vi "AutoMode.vi"(8 "error in (no error)":errorcluster, 11 "AutoModeData":T1) -> (0 "error out":errorcluster)   [LabVIEW 2019, in "AutoMode.lvlib"]
uses:
  AutoMode.lvlib
  Cluster - AutoModeData.ctl
  MainController/Cluster - TestSettings.ctl
  MainController/Cluster - HardwareConfiguration.ctl
  MainController/Cluster - TestResults.ctl
  Cluster - AutoModeMessage.ctl
  Enum - AutoModeState.ctl
  MainController/Cluster - MainControllerMessage.ctl
  MainController/Enum - MainState.ctl
  support/User Event - Stop/User Event - Stop.lvlib
  MainController/MainController.lvlib
panel:
  in  "Manual Return To Zero":bool=TRUE
  in  "Dwell Time":dbl min=0.0 step=1.0 format="%.2f s"
  in  "Auto Increment":bool=TRUE
  in  "AutoGenerate":bool
  in  "Output Data Path":path
  in  "Goto Zero":bool
  in  "Zero Position":bool
  out "TravelForce":cluster{"Travel":dbl, "Force":dbl, "Work":dbl} {"Work" format="%.3f"; "Force" format="%.3f"; "Travel" format="%.3f"}
  in  "Applicator Prefix":string="Applicator Test"
  in  "Sample":u32=1
  in  "Winding Speed":dbl min=0.0 step=1.0 format="%.2f °/s"
  in  "Winding Distance":dbl min=0.0 step=1.0 format="%.2f °"
  out "TestRuntime":i64 format="%<%H:%M:%S>t"
  out "XY Graph":T5(graph)
  out "Waveform":dbl[][](graph) caption="Waveform Chart"
  out "Work":cluster{dbl[], "Real Matrix":dbl[]}[](graph)
  out "Running":bool
  # "Test Settings"
  # "Commands"
  # "DAQ I/O"
  # "Test Runtime"
  # "Travel (deg)"
  # "Force (N)"
  # "Work"
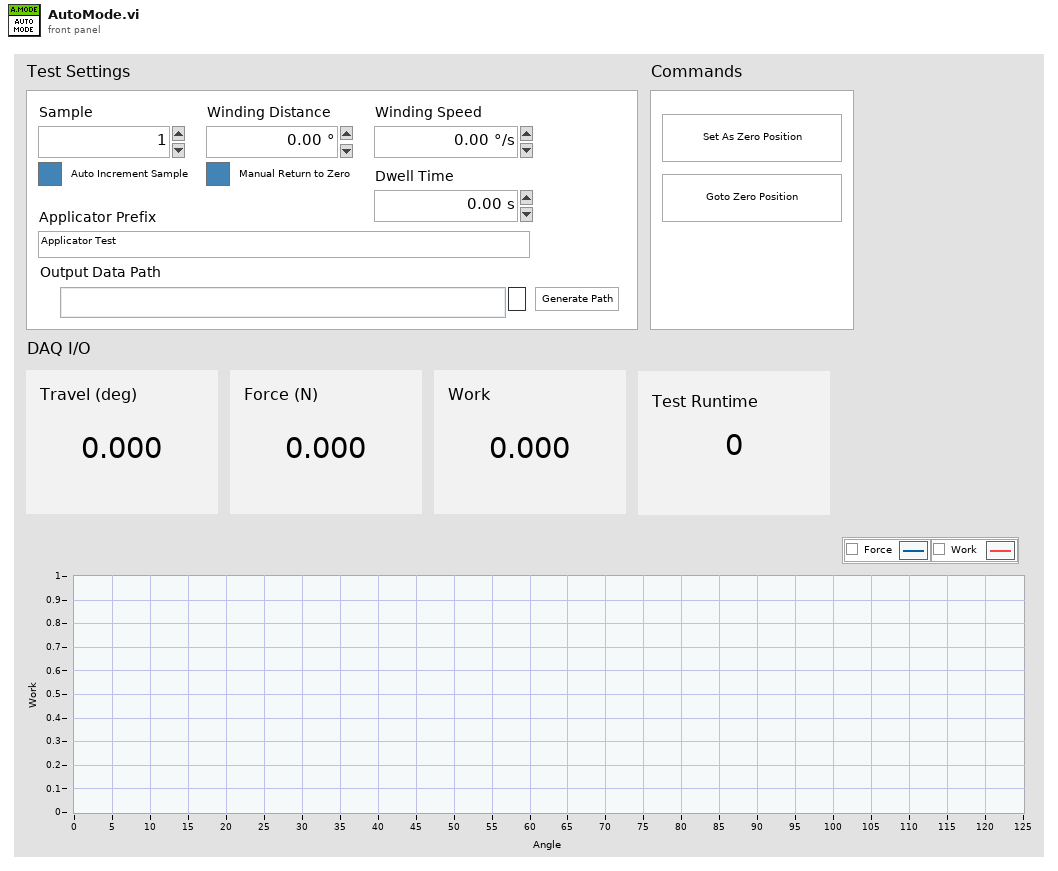
[diagram p1: front panel]
types:
  T1 = typedef "AutoMode.lvlib/Cluster - AutoModeData.ctl" = cluster{"DataDisplayQueue":refnum<queue>, "StepStartTime":timestamp, "TestSettings":T2, "Hardware Configuration":T3, "TestResults":T4, "ElapsedTime":dbl, "IsFirstSample":bool, "UIRefs":map{string, refnum<vi>}, "SelfQueue":refnum<queue>, "MainQueue":refnum<queue>}
  T2 = typedef "MainController.lvlib/Cluster - TestSettings.ctl" = cluster{"Sample":u32, "Applicator Prefix":string, "Winding Distance":dbl, "Winding Speed":dbl, "Dwell Time":dbl, "Auto Increment Sample":bool, "Output Data Path":path, "File Base Path":path, "Manual Return To Zero":bool}
  T3 = typedef "MainController.lvlib/Cluster - HardwareConfiguration.ctl" = cluster{"Mark10COM":refnum<visa-resource-name>, "IsConnected":bool}
  T4 = typedef "MainController.lvlib/Cluster - TestResults.ctl" = cluster{"AcquiredData":dbl[][], "TestStartTime":timestamp}
  T5 = cluster{"XY Graph":cluster{"X":dbl, "Y":dbl}[]}[]
  T6 = typedef "AutoMode.lvlib/Cluster - AutoModeMessage.ctl" = cluster{"Message":T7, "Data":variant}
  T7 = typedef "AutoMode.lvlib/Enum - AutoModeState.ctl" = enum16{"Initialize", "Idle", "UpdateConfig", "UpdateHWConfig", "BroadcastSettings", "Start", "CheckValidReportPath", "Winding", "WaitForWinding", "Unwind", "WaitForUnwind", "Stop", "Abort", "WriteDataToFile", "EventTriggered", "GenerateFilePath", "ZeroPosition", "GotoZero", "Error", "Exit"}
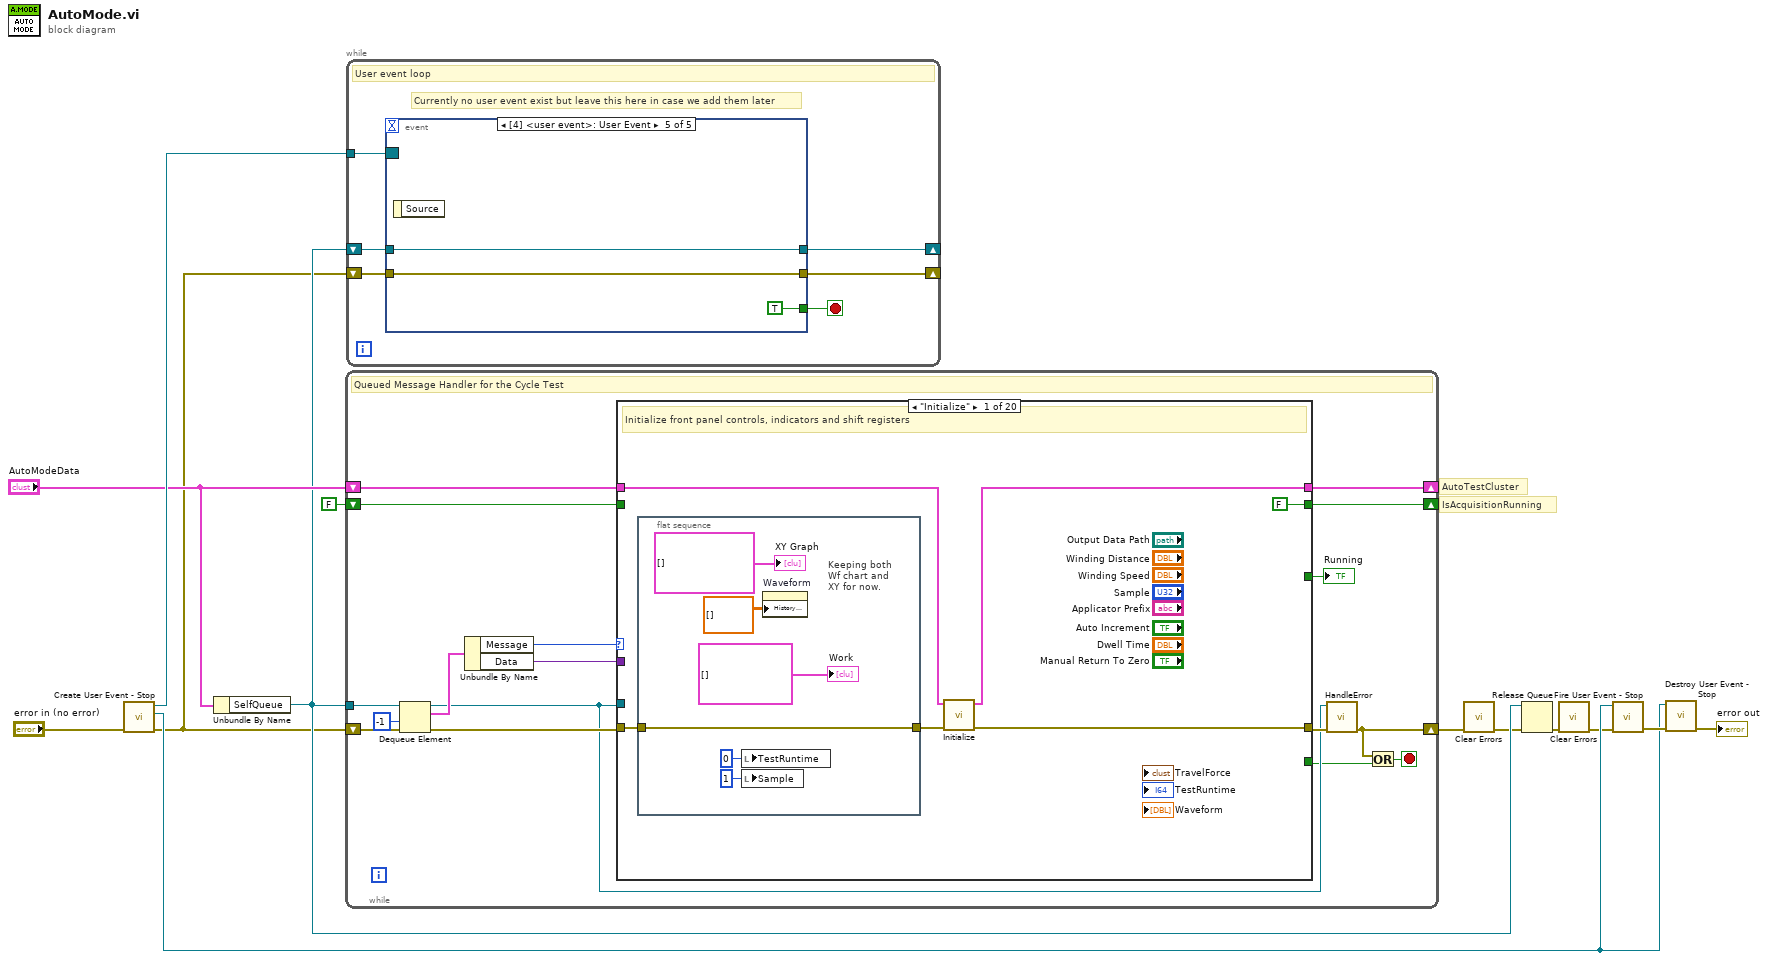
[diagram p0: block diagram]
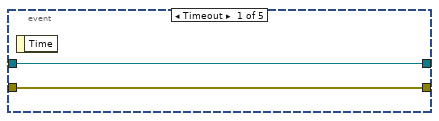
[diagram p2: hidden frame]
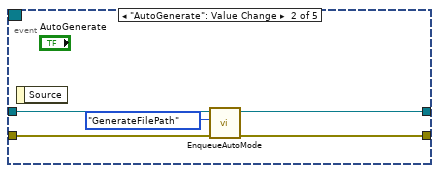
[diagram p3: hidden frame]
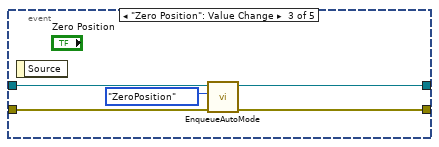
[diagram p4: hidden frame]
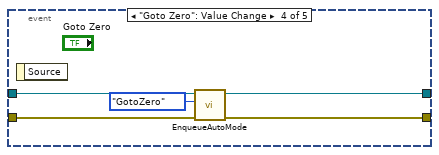
[diagram p5: hidden frame]
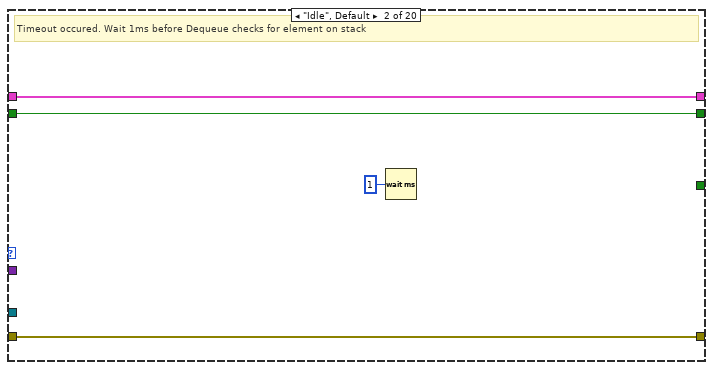
[diagram p6: hidden frame]
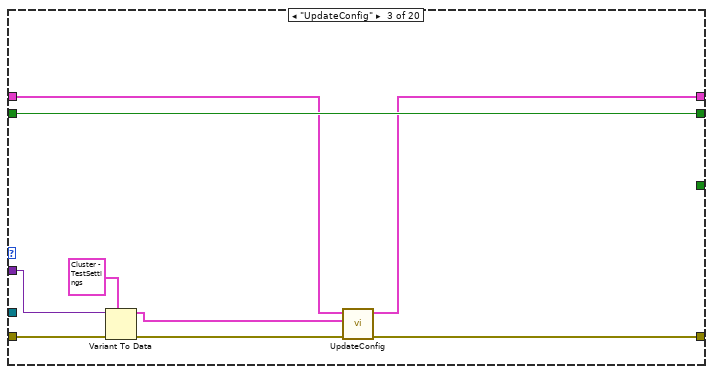
[diagram p7: hidden frame]
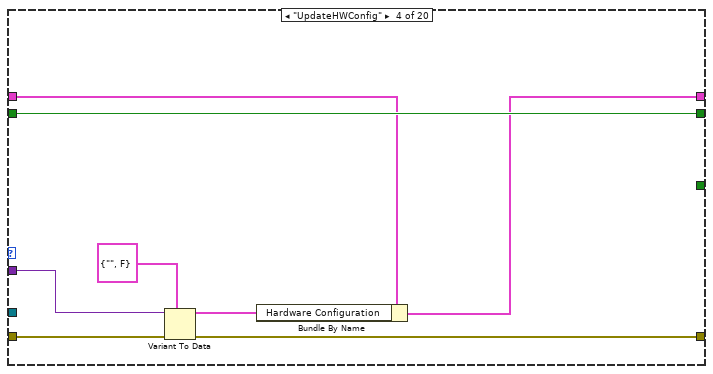
[diagram p8: hidden frame]
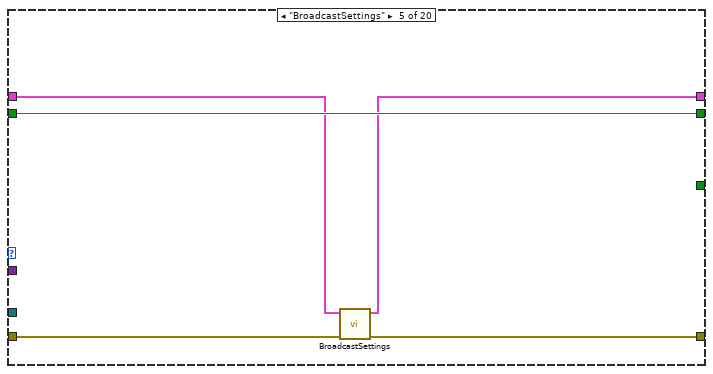
[diagram p9: hidden frame]
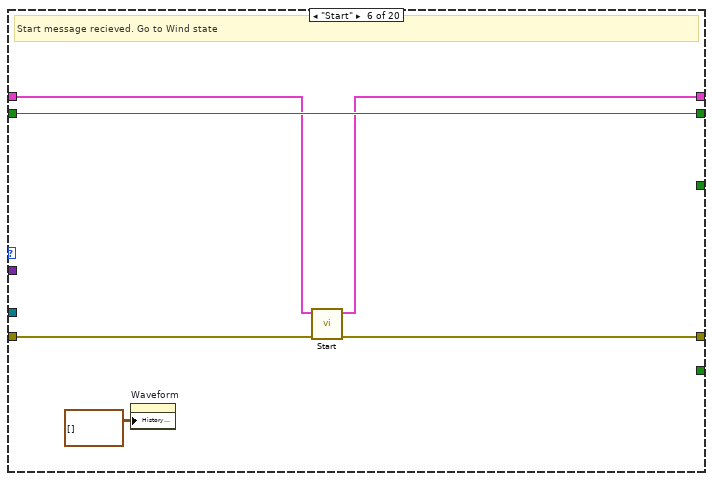
[diagram p10: hidden frame]
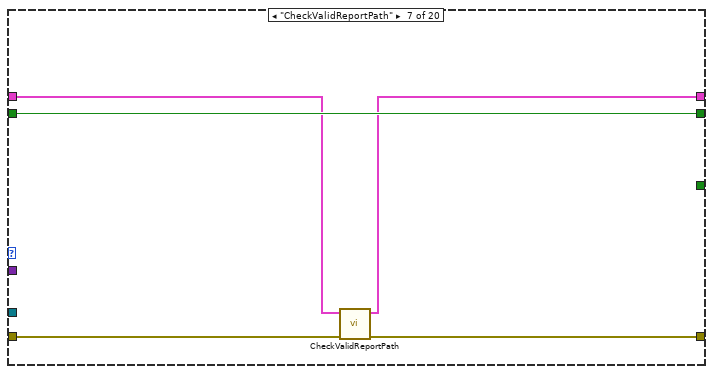
[diagram p11: hidden frame]
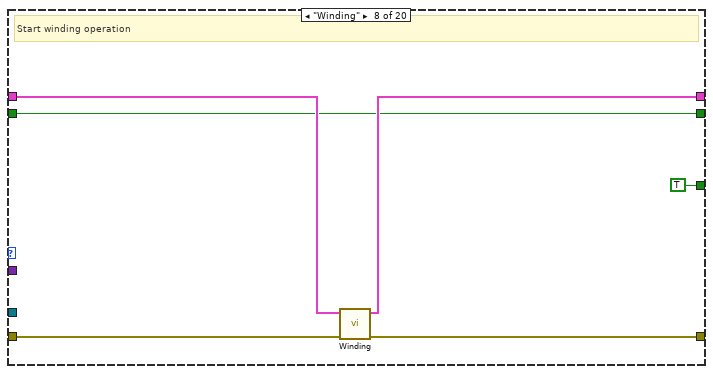
[diagram p12: hidden frame]
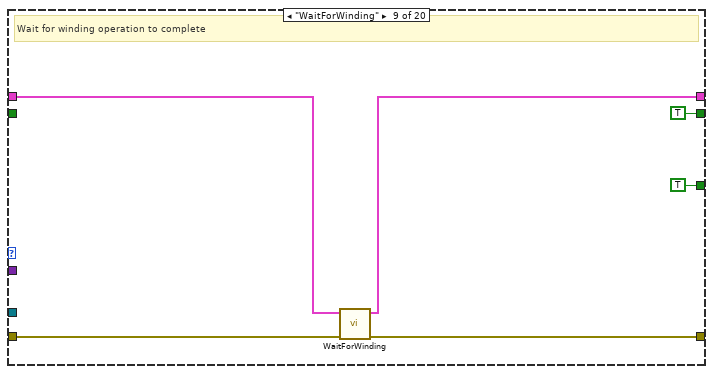
[diagram p13: hidden frame]
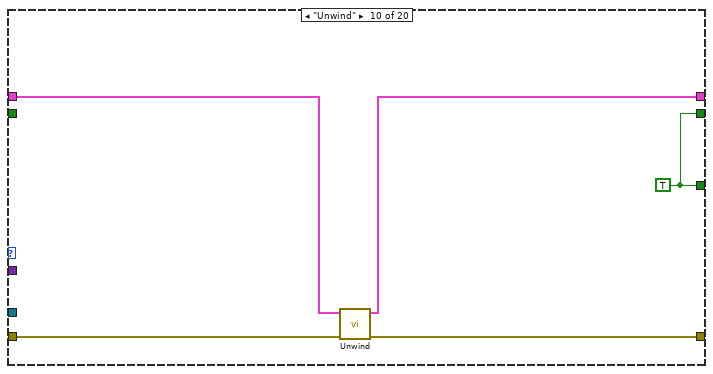
[diagram p14: hidden frame]
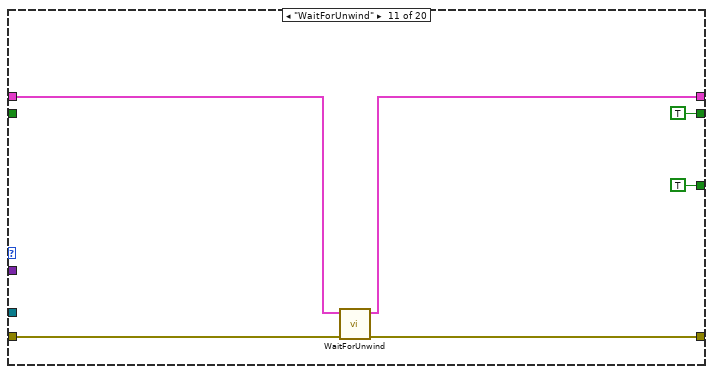
[diagram p15: hidden frame]
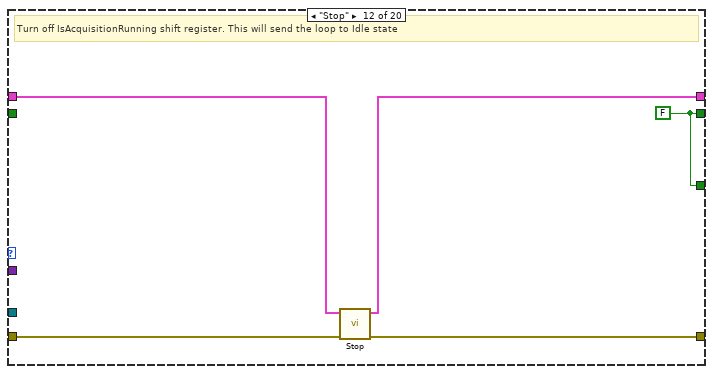
[diagram p16: hidden frame]
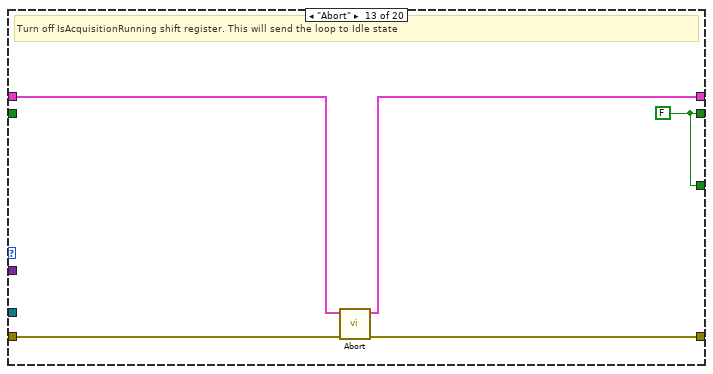
[diagram p17: hidden frame]
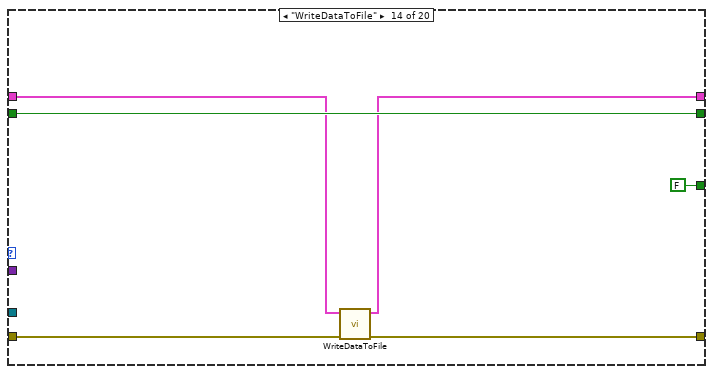
[diagram p18: hidden frame]
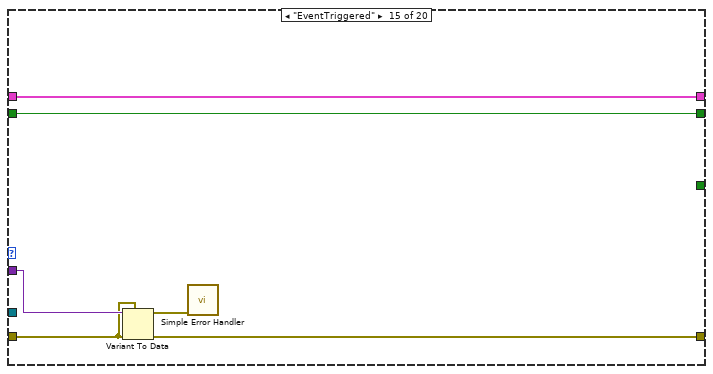
[diagram p19: hidden frame]
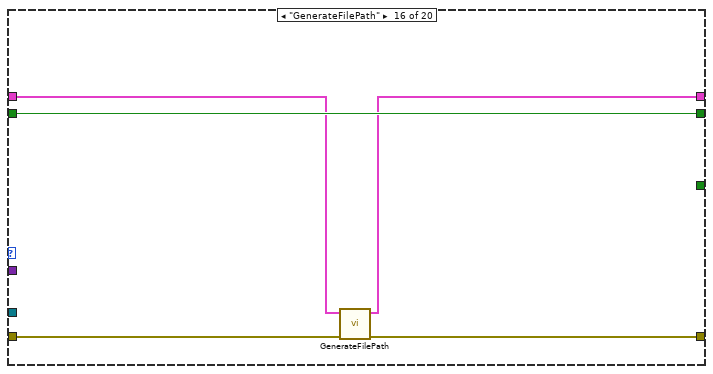
[diagram p20: hidden frame]
diagram:
  # "AutoTestCluster"
  # "IsAcquisitionRunning"
  n1 = call "Create User Event - Stop.vi"("error in (no error)"="error in (no error)") -> ("error out"=w3:errorcluster, "User Event - Stop"=w8:refnum<user-event>, "Stop Event Registration Refnum"=w12:refnum<event-registration>)  [unwired: 8 in]
  n2 = Unbundle By Name("AutoModeData") -> ("SelfQueue"=w4:refnum<queue>)
  n3 = while {
    tunnel: w4 -> [w29]
    shift-right: [w23] -> _
    shift-left: "AutoModeData" -> [w24]
    shift-right: [w21] -> _
    shift-left: FALSE -> [w20]
    shift-right: [w14] -> w13
    shift-left: w3 -> [w30]
    stop <- w15 stop-if-true
    # "Queued Message Handler for the Cycle Test"
    n4 = Dequeue Element(queue=w29, timeout in ms (-1)=-1, error in (no error)=w30) -> (queue out=w19:refnum<queue>, element=w28:T6, error out=w26:errorcluster)  [unwired: 1 out]
    n5 = Unbundle By Name(w28) -> ("Message"=w17:T7, "Data"=w25:variant)
    n6 = case shown="\"Initialize\"" w17 {
      tunnel: [w31 w43 w49 w61 w66 w71 w77 w83 w88 w94 w99 w105 w110 w115 w122 w127 w132 w137 w142 w153] -> w27
      tunnel: w26 -> [w32 w43 w55 w63 w67 w72 w78 w84 w89 w95 w100 w106 w111 w116 w120 w129 w133 w138 w146 w153]
      tunnel: [_ _ _ _ _ _ _ _ _ _ _ _ _ _ _ _ _ _ FALSE TRUE] -> w16
      tunnel: w25 -> [_ _ w52 w60 _ _ _ _ _ _ _ _ _ _ w121 _ _ _ w148 _]
      tunnel: w24 -> [w35 w46 w50 w56 w65 w70 w76 w82 w87 w93 w98 w104 w109 w114 w124 w126 w131 w136 w144 w152]
      tunnel: [w34 w46 w48 w57 w64 w69 w75 w81 w86 w92 w97 w103 w108 w113 w124 w125 w130 w135 w144 w152] -> w23
      tunnel: [_ _ _ _ _ _ _ TRUE TRUE w96 TRUE w107 w112 FALSE _ _ _ _ w140 _] -> w22
      tunnel: [FALSE w45 w54 w62 w68 w74 w79 w80 TRUE w96 TRUE w107 w112 w118 w123 w128 w134 w139 w140 w151] -> w21
      tunnel: w20 -> [_ w45 w54 w62 w68 w74 w79 w80 _ _ _ _ _ w118 w123 w128 w134 w139 _ w151]
      tunnel: w19 -> [_ _ _ _ _ _ _ _ _ _ _ _ _ _ _ _ _ _ _ _]
      frame "Initialize" {
        # "Initialize front panel controls, indicators and shift registers"
        n7 = flat-sequence {
          tunnel: [w39] -> w33
          tunnel: w32 -> [w39]
          frame #0 {
            # "Keeping both\nWf chart and\nXY for now."
            n8 = local write "TestRuntime"(i64 0 ("TestRuntime")) -> ()
            n9 = local write "Sample"(u32 1 ("Sample")) -> ()
            n10 = property on="Waveform" class="WFChart (strict)"("History Data"=dbl[][] []) -> ()  [unwired: 2 in, 2 out]
            "Work" <- cluster{dbl[], "Real Matrix":dbl[]}[] [] ("LC-X vs Time")
            "XY Graph" <- T5 [] ("appended array")
          }
        }
        n11 = call "Initialize.vi"("Error In"=w33, "AutoData"=w35) -> ("Error Out"=w31:errorcluster, "AutoData out"=w34:T1)  [unwired: 8 in]
      }
      frame "Idle", Default {
        # "Timeout occured. Wait 1ms before Dequeue checks for element on stack"
        n12 = Wait (ms)(milliseconds to wait=u32 1) -> ()  [unwired: 1 out]
      }
      frame "UpdateConfig" {
        n13 = Variant To Data(error in=w55, type=T2 {"Sample"=0, "Applicator Prefix"="", "Winding Distance"=0.0, "Winding Speed"=0.0, "Dwell Time"=0.0, "Auto Increment Sample"=FALSE, "Output Data Path"=path "", "File Base Path"=path "", "Manual Return To Zero"=FALSE} ("TestSettings"), Variant=w52) -> (data=w47:T2, error out=w53:errorcluster)
        n14 = call "UpdateConfig.vi"("Error In"=w53, "TestSettings"=w47, "AutoData"=w50) -> ("Error Out"=w49:errorcluster, "AutoData out"=w48:T1)  [unwired: 7 in]
      }
      frame "UpdateHWConfig" {
        n15 = Variant To Data(error in=w63, type=T3 {"Mark10COM"="", "IsConnected"=FALSE} ("HardwareConfig"), Variant=w60) -> (data=w58:T3, error out=w61:errorcluster)
        n16 = Bundle By Name(cluster=w56, "Hardware Configuration"=w58) -> (w57:T1)
      }
      frame "BroadcastSettings" {
        n17 = call "BroadcastSettings.vi"("Error In"=w67, "AutoData"=w65) -> ("Error Out"=w66:errorcluster, "AutoData out"=w64:T1)  [unwired: 8 in]
      }
      frame "Start" {
        # "Start message recieved. Go to Wind state"
        n18 = property on="Waveform" class="WFChart (strict)"("History Data"=waveform(dbl)[][] []) -> ()  [unwired: 2 in, 2 out]
        n19 = call "Start.vi"("Error In"=w72, "AutoData"=w70) -> ("Error Out"=w71:errorcluster, "AutoData out"=w69:T1)  [unwired: 8 in]
      }
      frame "CheckValidReportPath" {
        n20 = call "CheckValidReportPath.vi"("Error In"=w78, "AutoData"=w76) -> ("Error Out"=w77:errorcluster, "AutoData out"=w75:T1)  [unwired: 8 in]
      }
      frame "Winding" {
        # "Start winding operation"
        n21 = call "Winding.vi"("Error In"=w84, "AutoData"=w82) -> ("Error Out"=w83:errorcluster, "AutoData out"=w81:T1)  [unwired: 8 in]
      }
      frame "WaitForWinding" {
        # "Wait for winding operation to complete"
        n22 = call "WaitForWinding.vi"("Error In"=w89, "AutoData"=w87) -> ("Error Out"=w88:errorcluster, "AutoData out"=w86:T1)  [unwired: 8 in]
      }
      frame "Unwind" {
        w96 = TRUE
        n23 = call "Unwind.vi"("Error In"=w95, "AutoData"=w93) -> ("Error Out"=w94:errorcluster, "AutoData out"=w92:T1)  [unwired: 8 in]
      }
      frame "WaitForUnwind" {
        n24 = call "WaitForUnwind.vi"("Error In"=w100, "AutoData"=w98) -> ("Error Out"=w99:errorcluster, "AutoData out"=w97:T1)  [unwired: 8 in]
      }
      frame "Stop" {
        w107 = FALSE
        # "Turn off IsAcquisitionRunning shift register. This will send the loop to Idle state"
        n25 = call "Stop.vi"("Error In"=w106, "AutoData"=w104) -> ("Error Out"=w105:errorcluster, "AutoData out"=w103:T1)  [unwired: 8 in]
      }
      frame "Abort" {
        w112 = FALSE
        # "Turn off IsAcquisitionRunning shift register. This will send the loop to Idle state"
        n26 = call "Abort.vi"("Error In"=w111, "AutoData"=w109) -> ("Error Out"=w110:errorcluster, "AutoData out"=w108:T1)  [unwired: 8 in]
      }
      frame "WriteDataToFile" {
        n27 = call "WriteDataToFile.vi"("Error In"=w116, "AutoData"=w114) -> ("Error Out"=w115:errorcluster, "AutoData out"=w113:T1)  [unwired: 8 in]
      }
      frame "EventTriggered" {
        n28 = Variant To Data(error in=w120, type=w120, Variant=w121) -> (data=w119:errorcluster, error out=w122:errorcluster)
        n29 = call <vilib>:"Simple Error Handler.vi"("error in (no error)"=w119) -> ()  [unwired: 4 in, 5 out]
      }
      frame "GenerateFilePath" {
        n30 = call "GenerateFilePath.vi"("Error In"=w129, "AutoData"=w126) -> ("Error Out"=w127:errorcluster, "AutoData out"=w125:T1)  [unwired: 8 in]
      }
      frame "ZeroPosition" {
        n31 = call "ZeroPosition.vi"("Error In"=w133, "AutoData"=w131) -> ("Error Out"=w132:errorcluster, "AutoData out"=w130:T1)  [unwired: 8 in]
      }
      frame "GotoZero" {
        n32 = call "GotoZero.vi"("Error In"=w138, "AutoData"=w136) -> ("Error Out"=w137:errorcluster, "AutoData out"=w135:T1)  [unwired: 8 in]
      }
      frame "Error" {
        w140 = FALSE
        n33 = Variant To Data(error in=w146, type=errorcluster {"status"=FALSE, "code"=0, "source"=""} ("error out"), Variant=w148) -> (data=w145:errorcluster)  [unwired: 1 out]
        n34 = Unbundle By Name(w144) -> ("MainQueue"=w143:refnum<queue>)
        n35 = call "ForwardErrorToCaller.vi"("error in (no error)"=w145, "Main"=w143) -> ("error out"=w141:errorcluster)  [unwired: 9 in]
        n36 = Merge Errors(w141, w146) -> (w142:errorcluster)
      }
      frame "Exit" {
      }
    }
    "Running" <- w22
    n37 = call "HandleError.vi"("error in (no error)"=w27, "Queue in"=w19) -> ("error out"=w14:errorcluster)  [unwired: 8 in, 1 out]
    n38 = Or(x=w14, y=w16) -> (x .or. y?=w15:bool)
  }
  n39 = while {
    tunnel: w12 -> [w159]
    shift-right: [w155] -> _
    shift-left: w3 -> [w156]
    shift-right: [w154] -> _
    shift-left: w4 -> [w158]
    stop <- w157 stop-if-true
    # "Currently no user event exist but leave this here in case we add them later"
    # "User event loop"
    n40 = event shown="[4] <user event>: User Event" {
      selector: w159 -> [_ _ _ _ _]
      dyn-events: _ -> [_ _ _ _ _]
      timeout: _ -> [_ _ _ _ _]
      tunnel: w158 -> [w160 w166 w171 w176 w177]
      tunnel: [_ _ _ _ TRUE] -> w157
      tunnel: w156 -> [w161 w163 w169 w174 w178]
      tunnel: [w161 w164 w168 w173 w178] -> w155
      tunnel: [w160 w162 w167 w172 w177] -> w154
      event Timeout {
        n41 = event-data() -> ()  [unwired: 1 in, 1 out]
      }
      event "AutoGenerate": Value Change {
        n42 = event-data() -> ()  [unwired: 1 in, 1 out]
        n43 = call "EnqueueAutoMode.vi"("error in (no error)"=w163, "AutoState"=Enum_-_AutoModeState."GenerateFilePath" ("CycleTestState"), "Queue in"=w166) -> ("error out"=w164:errorcluster, "queue out"=w162:refnum<queue>)  [unwired: 7 in]
      }
      event "Zero Position": Value Change {
        n44 = event-data() -> ()  [unwired: 1 in, 1 out]
        n45 = call "EnqueueAutoMode.vi"("error in (no error)"=w169, "AutoState"=Enum_-_AutoModeState."ZeroPosition" ("CycleTestState"), "Queue in"=w171) -> ("error out"=w168:errorcluster, "queue out"=w167:refnum<queue>)  [unwired: 7 in]
      }
      event "Goto Zero": Value Change {
        n46 = event-data() -> ()  [unwired: 1 in, 1 out]
        n47 = call "EnqueueAutoMode.vi"("error in (no error)"=w174, "AutoState"=Enum_-_AutoModeState."GotoZero", "Queue in"=w176) -> ("error out"=w173:errorcluster, "queue out"=w172:refnum<queue>)  [unwired: 7 in]
      }
      event User Event {
        n48 = event-data() -> ()  [unwired: 1 in, 1 out]
      }
    }
  }
  n49 = call <vilib>:"Clear Errors.vi"("error in (no error)"=w13) -> ("error out"=w2:errorcluster)  [unwired: 5 in, 1 out]
  n50 = Release Queue(queue=w4, error in (no error)=w2) -> (error out=w11:errorcluster)  [unwired: 1 in, 2 out]
  n51 = call <vilib>:"Clear Errors.vi"("error in (no error)"=w11) -> ("error out"=w1:errorcluster)  [unwired: 5 in, 1 out]
  n52 = call "Fire User Event - Stop.vi"("error in (no error)"=w1, "User Event - Stop"=w8) -> ("error out"=w9:errorcluster)  [unwired: 9 in]
  n53 = call "Destroy User Event - Stop.vi"("error in (no error)"=w9, "User Event - Stop"=w8) -> ("error out"=→"error out":errorcluster)  [unwired: 9 in]
